vi "BinarySearch2.vi"(4 "ExistingWts 1D Array":dbl[](array[numeric]), 6 "Exception List":csg[](array[numeric]), 8 "Desired Angle (degrees)":dbl, 9 "Desired Weight":dbl, 10 "Angles 1D Array":dbl[](array[numeric]), 11 "Weights 1D Array":dbl[](array[numeric])) -> (0 "Closest Angle 2":dbl, 1 "Closest Weight 2":dbl, 2 "Closest Angle 1":dbl, 3 "Closest Weight 1":dbl)   [LabVIEW 2012]
panel:
  out "Numeric":dbl
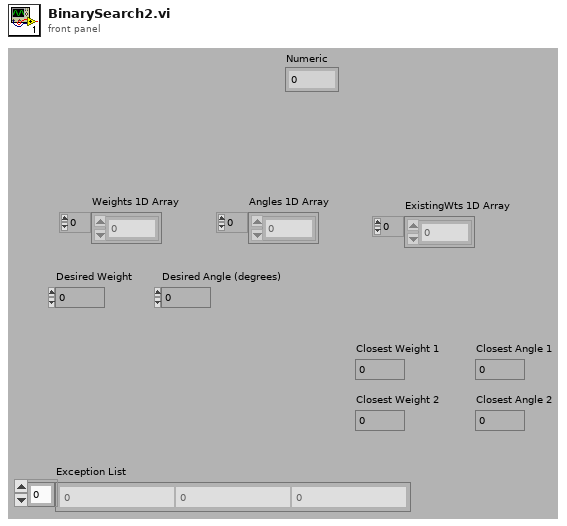
[diagram p1: front panel]
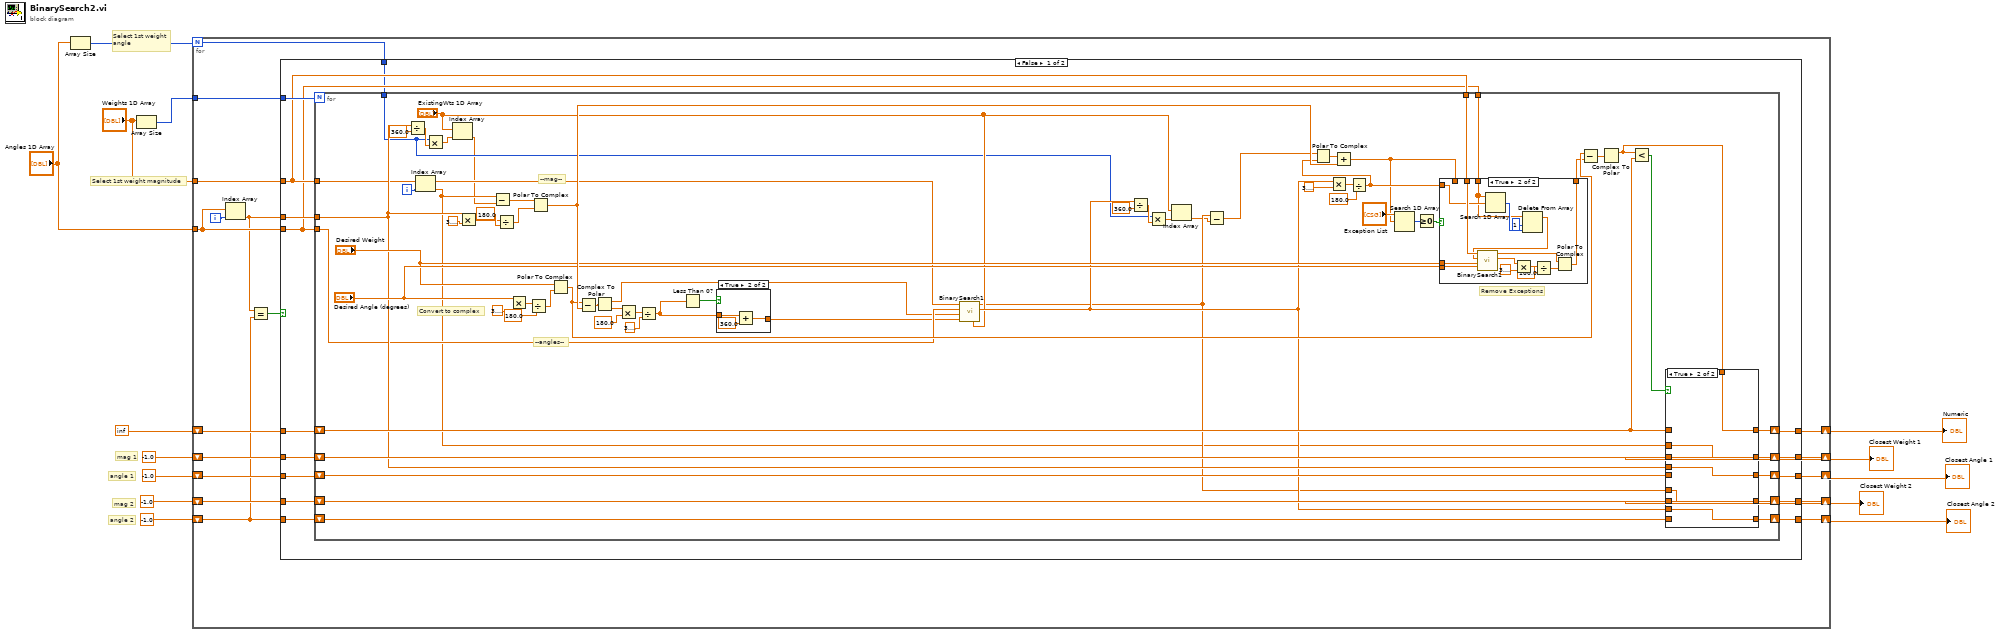
[diagram p0: block diagram]
diagram:
  # "Select 1st weight magnitude"
  # "Select 1st weight\nangle"
  # "angle 2"
  # "angle 1"
  # "mag 2"
  # "mag 1"
  n1 = Array Size(array="Angles 1D Array") -> (size(s)=w2:i32)
  n2 = Array Size(array="Weights 1D Array") -> (size(s)=w1:i32)
  n3 = for {
    N: w2 -> [w16]
    tunnel: w1 -> [w31]
    tunnel: "Weights 1D Array" -> [w29]
    tunnel: "Angles 1D Array" -> [w18]
    shift-right: [w22] -> w3
    shift-left: inf -> [w21]
    shift-right: [w26] -> w4
    shift-left: -1.0 -> [w28]
    shift-right: [w25] -> w5
    shift-left: -1.0 -> [w27]
    shift-right: [w24] -> w6
    shift-left: -1.0 -> [w20]
    shift-right: [w23] -> w7
    shift-left: -1.0 -> [w15]
    i -> [w30]
    n4 = Index Array(array=w18, index=w30) -> (element=w17:dbl)
    n5 = Equal?(x=w17, y=w15) -> (x = y?=w19:bool)
    n6 = case shown="False" w19 {
      tunnel: w31 -> [w46 _]
      tunnel: w17 -> [w45 _]
      tunnel: w29 -> [w34 _]
      tunnel: w18 -> [w33 _]
      tunnel: w28 -> [w44 w145]
      tunnel: w27 -> [w43 w144]
      tunnel: w20 -> [w42 w143]
      tunnel: w15 -> [w41 w142]
      tunnel: [w40 w145] -> w26
      tunnel: [w39 w144] -> w25
      tunnel: [w38 w143] -> w24
      tunnel: [w37 w142] -> w23
      tunnel: [w36 w146] -> w22
      tunnel: w21 -> [w35 w146]
      tunnel: w16 -> [w32 _]
      frame False {
        n7 = for {
          N: w46 -> [_]
          tunnel: w45 -> [w64]
          tunnel: w33 -> [w62]
          tunnel: w34 -> [w58]
          shift-right: [w103] -> w40
          shift-left: w44 -> [w102]
          shift-right: [w101] -> w39
          shift-left: w43 -> [w100]
          shift-right: [w98] -> w38
          shift-left: w42 -> [w99]
          shift-right: [w97] -> w37
          shift-left: w41 -> [w96]
          shift-right: [w105] -> w36
          shift-left: w35 -> [w104]
          tunnel: w34 -> [w78]
          tunnel: w33 -> [w77]
          tunnel: w32 -> [w51]
          i -> [w111]
          # "Remove Exceptions"
          # "--angles--"
          # "--mag--"
          # "Convert to complex"
          n8 = Divide(x=w64, y=360.0) -> (x/y=w66:dbl)
          n9 = Index Array(array=w58, index=w111) -> (element=w48:dbl)
          n10 = Multiply(x=w51, y=w66) -> (x*y=w65:dbl)
          n11 = Index Array(array="ExistingWts 1D Array", index=w65) -> (element=w47:dbl)
          n12 = Multiply(x=w64, y=3.141592653589793) -> (x*y=w68:dbl)
          n13 = Subtract(x=w48, y=w47) -> (x-y=w59:dbl)
          n14 = Divide(x=w68, y=180.0) -> (x/y=w67:dbl)
          n15 = Multiply(x="Desired Angle (degrees)", y=3.141592653589793) -> (x*y=w94:dbl)
          n16 = Divide(x=w94, y=180.0) -> (x/y=w92:dbl)
          n17 = Polar To Complex(1:w67, 2:w59) -> (0:w108:cdb)
          n18 = Polar To Complex(1:w92, 2:"Desired Weight") -> (0:w76:cdb)
          n19 = Subtract(x=w76, y=w108) -> (x-y=w110:cdb)
          n20 = Complex To Polar(r * e^(i*theta)=w110) -> (r=w61:dbl, theta=w90:dbl)
          n21 = Multiply(x=w90, y=180.0) -> (x*y=w91:dbl)
          n22 = Divide(x=w91, y=3.141592653589793) -> (x/y=w83:dbl)
          n23 = Less Than 0?(x=w83) -> (x < 0?=w84:bool)
          n24 = case shown="True" w84 {
            tunnel: w83 -> [w128 w131]
            tunnel: [w128 w129] -> w60
            frame False {
            }
            frame True {
              n25 = Add(x=w131, y=360.0) -> (x+y=w129:dbl)
            }
          }
          n26 = call "BinarySearch1.vi"("ExistingWts 1D Array"="ExistingWts 1D Array", "Desired Angle (degrees)"=w60, "Desired Weight"=w61, "Angles 1D Array"=w62, "Weights 1D Array"=w58) -> ("Closest Angle 1"=w55:dbl, "Closest Weight 1"=w50:dbl)  [unwired: 5 in]
          n27 = Divide(x=w55, y=360.0) -> (x/y=w56:dbl)
          n28 = Multiply(x=w51, y=w56) -> (x*y=w54:dbl)
          n29 = Index Array(array="ExistingWts 1D Array", index=w54) -> (element=w49:dbl)
          n30 = Subtract(x=w50, y=w49) -> (x-y=w52:dbl)
          n31 = Multiply(x=w55, y=3.141592653589793) -> (x*y=w87:dbl)
          n32 = Divide(x=w87, y=180.0) -> (x/y=w73:dbl)
          n33 = Polar To Complex(1:w73, 2:w52) -> (0:w109:cdb)
          n34 = Add(x=w109, y=w108) -> (x+y=w71:cdb)
          n35 = Search 1D Array(1D array="Exception List", element=w71) -> (index of element=w80:i32)  [unwired: 1 in]
          n36 = Greater Or Equal To 0?(x=w80) -> (x >= 0?=w79:bool)
          n37 = case shown="True" w79 {
            tunnel: w78 -> [_ w127]
            tunnel: w77 -> [_ w121]
            tunnel: "Desired Angle (degrees)" -> [_ w125]
            tunnel: "Desired Weight" -> [_ w126]
            tunnel: w73 -> [_ w124]
            tunnel: [w112 w113] -> w72
            tunnel: w71 -> [w112 _]
            frame False {
            }
            frame True {
              n38 = Search 1D Array(1D array=w121, element=w124) -> (index of element=w123:i32)  [unwired: 1 in]
              n39 = Delete From Array(array=w121, length=1, index=w123) -> (array with subset deleted=w120:dbl[])  [unwired: 1 out]
              n40 = call "BinarySearch1.vi"("Desired Angle (degrees)"=w125, "Desired Weight"=w126, "Angles 1D Array"=w120, "Weights 1D Array"=w127) -> ("Closest Angle 1"=w117:dbl, "Closest Weight 1"=w118:dbl)  [unwired: 6 in]
              n41 = Multiply(x=w117, y=3.141592653589793) -> (x*y=w119:dbl)
              n42 = Divide(x=w119, y=180.0) -> (x/y=w114:dbl)
              n43 = Polar To Complex(1:w114, 2:w118) -> (0:w113:cdb)
            }
          }
          n44 = Subtract(x=w76, y=w72) -> (x-y=w107:cdb)
          n45 = Complex To Polar(r * e^(i*theta)=w107) -> (r=w106:dbl)  [unwired: 1 out]
          n46 = Less?(x=w106, y=w104) -> (x < y?=w82:bool)
          n47 = case shown="True" w82 {
            tunnel: w104 -> [w136 _]
            tunnel: [w136 w141] -> w105
            tunnel: w106 -> [_ w141]
            tunnel: [w135 w139] -> w103
            tunnel: w102 -> [w135 _]
            tunnel: [w134 w138] -> w101
            tunnel: w100 -> [w134 _]
            tunnel: w99 -> [w133 _]
            tunnel: [w133 w137] -> w98
            tunnel: [w132 w140] -> w97
            tunnel: w96 -> [w132 _]
            tunnel: w50 -> [_ w137]
            tunnel: w55 -> [_ w140]
            tunnel: w48 -> [_ w139]
            tunnel: w64 -> [_ w138]
            frame False {
            }
            frame True {
            }
          }
        }
      }
      frame True {
      }
    }
  }
  "Closest Weight 1" <- w4
  "Closest Angle 1" <- w5
  "Closest Weight 2" <- w6
  "Closest Angle 2" <- w7
  "Numeric" <- w3
